vi "Material-Glue-Tree-AddSymbols.vi"(8 "error in (no error)":errorcluster, 11 "TreeControl in":refnum<vi>) -> (0 "error out":errorcluster, 3 "TreeControl out":refnum<vi>)   [LabVIEW 2013]
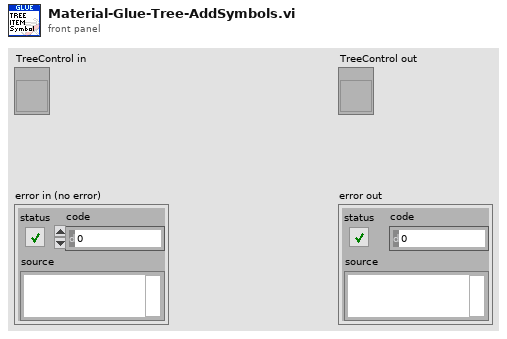
[diagram p1: front panel]
types:
  T1 = typedef "imagedata.ctl" = cluster{"image type":i32, "image depth":i32, "image":u8[], "mask":u8[], "colors":u32[], "Rectangle":cluster{"left":i16, "top":i16, "right":i16, "bottom":i16}}
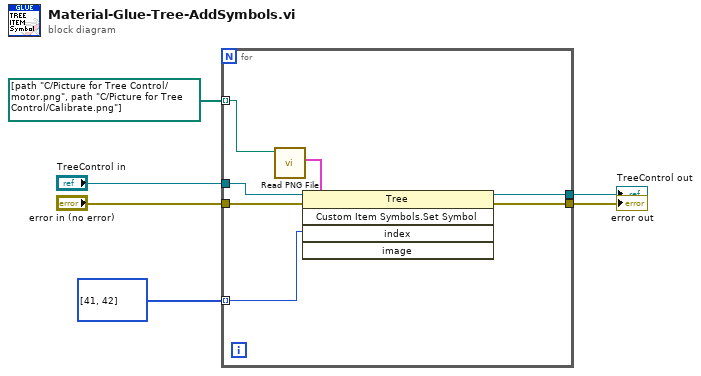
[diagram p0: block diagram]
diagram:
  n1 = for {
    tunnel: "error in (no error)" -> [w12]
    tunnel: [w11] -> w5
    tunnel: [w10] -> w4
    tunnel: "TreeControl in" -> [w9]
    tunnel: path[] [path "C:/Picture for Tree Control/motor.png", path "C:/Picture for Tree Control/Calibrate.png"] -> [w8] mode=indexing
    tunnel: i32[] [41, 42] -> [w7] mode=indexing
    n2 = call <vilib>:"Read PNG File.vi"("path to PNG file"=w8) -> ("image data"=w13:T1)  [unwired: 8 in, 2 out]
    n3 = invoke class="Tree" method="Custom Item Symbols.Set Symbol"(reference=w9, error in=w12, "index"=w7, "image"=w13) -> (reference out=w10:refnum<vi>, error out=w11:errorcluster)  [unwired: 1 in, 3 out]
  }
  "error out" <- w5
  "TreeControl out" <- w4
